vi "Control_giro_v2.vi"() -> ()   [LabVIEW 2025]
panel:
  in  "Boolean":bool
  out "Pulsos":dbl
  in  "B":bool
  in  "A":bool
  in  "stop":bool
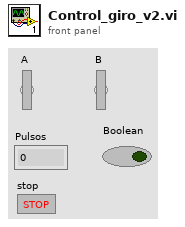
[diagram p1: front panel]
types:
  T1 = enum16{"Ini", "H1", "H2", "H3", "RES", "A1", "A2", "A3", "SUM"}
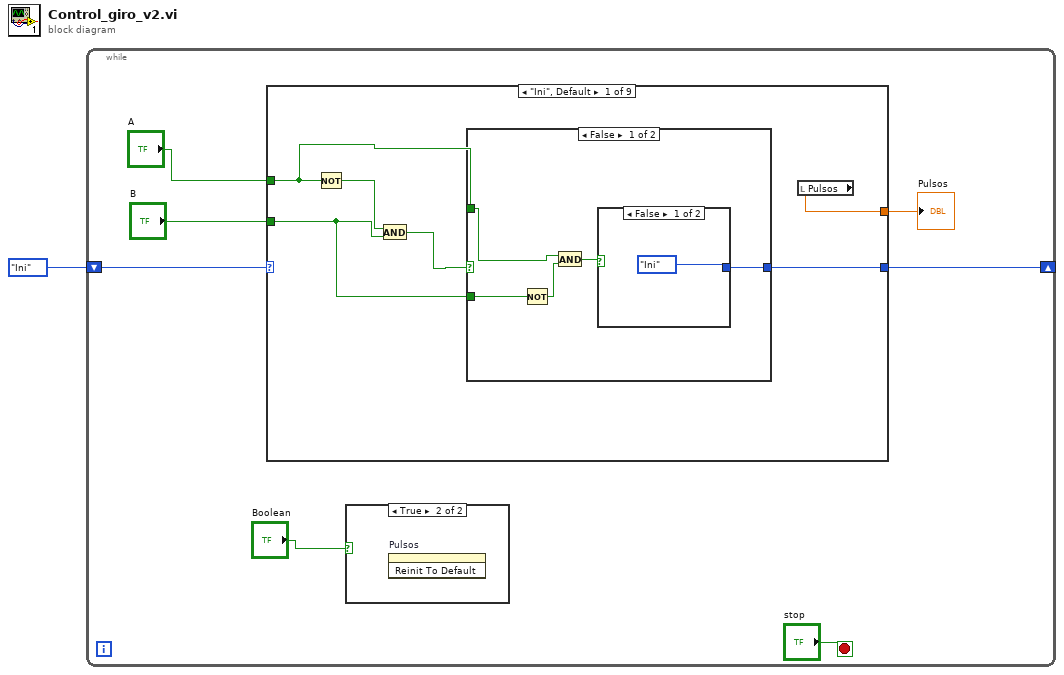
[diagram p0: block diagram]
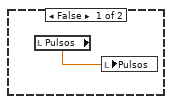
[diagram p2: hidden frame]
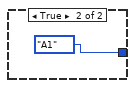
[diagram p3: hidden frame]
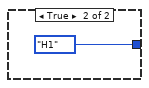
[diagram p4: hidden frame]
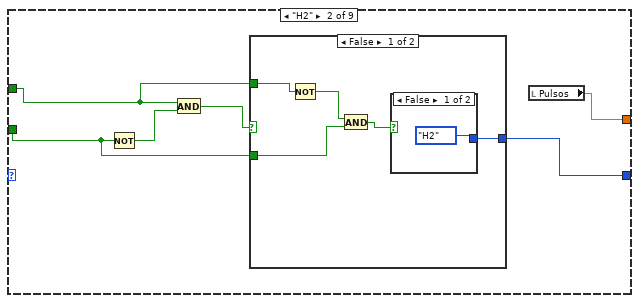
[diagram p5: hidden frame]
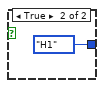
[diagram p6: hidden frame]
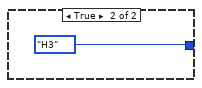
[diagram p7: hidden frame]
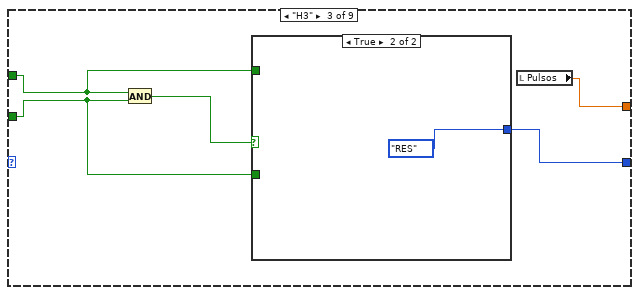
[diagram p8: hidden frame]
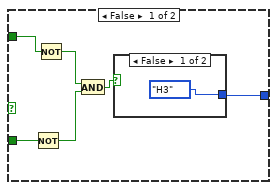
[diagram p9: hidden frame]
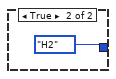
[diagram p10: hidden frame]
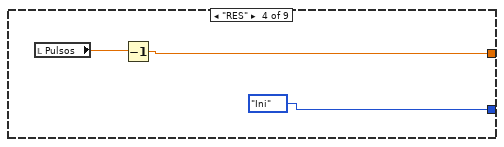
[diagram p11: hidden frame]
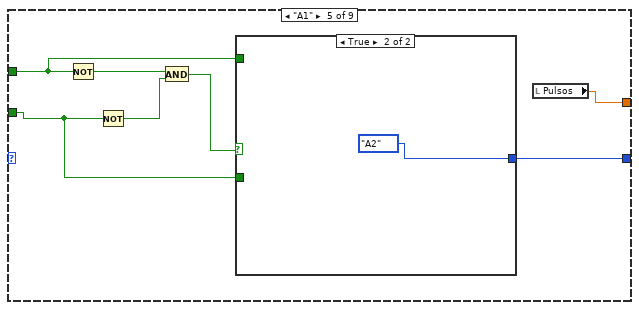
[diagram p12: hidden frame]
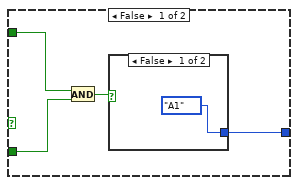
[diagram p13: hidden frame]
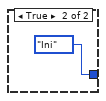
[diagram p14: hidden frame]
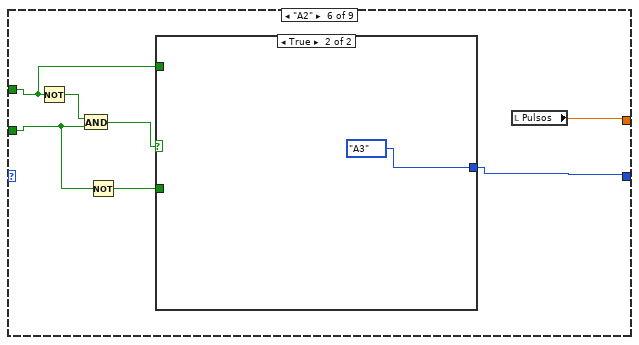
[diagram p15: hidden frame]
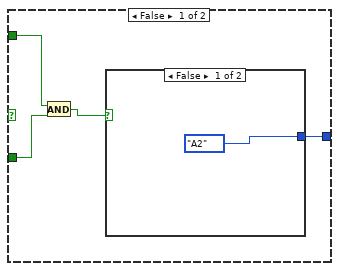
[diagram p16: hidden frame]
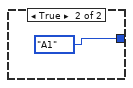
[diagram p17: hidden frame]
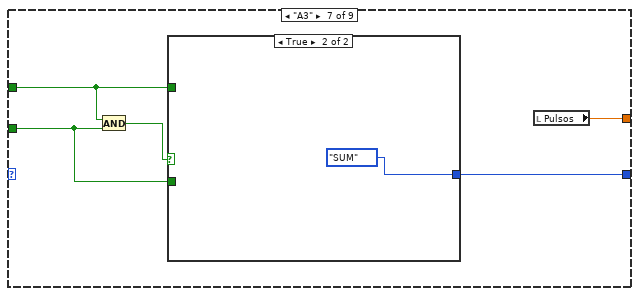
[diagram p18: hidden frame]
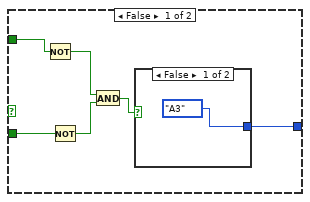
[diagram p19: hidden frame]
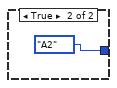
[diagram p20: hidden frame]
diagram:
  n1 = while {
    shift-right: [w4] -> _
    shift-left: T1."Ini" -> [w7]
    stop <- "stop" stop-if-true
    n2 = case shown="\"Ini\", Default" w7 {
      tunnel: "A" -> [w10 w27 w40 _ w57 w72 w84 _ w102]
      tunnel: "B" -> [w13 w26 w39 _ w56 w73 w85 _ w101]
      tunnel: [w14 w25 w41 T1."Ini" w58 w70 w86 T1."Ini" w103] -> w4
      tunnel: [w11 w24 w38 w53 w55 w69 w83 w98 w100] -> w3
      frame "Ini", Default {
        n3 = Not(x=w10) -> (.not. x?=w12:bool)
        n4 = And(x=w12, y=w13) -> (x .and. y?=w15:bool)
        n5 = case shown="False" w15 {
          tunnel: [w16 T1."H1"] -> w14
          tunnel: w13 -> [w20 _]
          tunnel: w10 -> [w19 _]
          frame False {
            n6 = Not(x=w20) -> (.not. x?=w18:bool)
            n7 = And(x=w19, y=w18) -> (x .and. y?=w17:bool)
            n8 = case shown="False" w17 {
              tunnel: [T1."Ini" T1."A1"] -> w16
              frame False {
              }
              frame True {
              }
            }
          }
          frame True {
          }
        }
        n9 = local read "Pulsos"() -> (w11:dbl)
      }
      frame "H2" {
        n10 = Not(x=w26) -> (.not. x?=w29:bool)
        n11 = And(x=w27, y=w29) -> (x .and. y?=w28:bool)
        n12 = case shown="False" w28 {
          tunnel: w27 -> [w34 _]
          tunnel: w26 -> [w33 _]
          tunnel: [w30 T1."H3"] -> w25
          frame False {
            n13 = Not(x=w34) -> (.not. x?=w32:bool)
            n14 = And(x=w32, y=w33) -> (x .and. y?=w31:bool)
            n15 = case shown="False" w31 {
              tunnel: [T1."H2" T1."H1"] -> w30
              frame False {
              }
              frame True {
              }
            }
          }
          frame True {
          }
        }
        n16 = local read "Pulsos"() -> (w24:dbl)
      }
      frame "H3" {
        n17 = And(x=w40, y=w39) -> (x .and. y?=w42:bool)
        n18 = case shown="True" w42 {
          tunnel: [w43 T1."RES"] -> w41
          tunnel: w40 -> [w48 _]
          tunnel: w39 -> [w47 _]
          frame False {
            n19 = Not(x=w47) -> (.not. x?=w44:bool)
            n20 = Not(x=w48) -> (.not. x?=w45:bool)
            n21 = And(x=w45, y=w44) -> (x .and. y?=w46:bool)
            n22 = case shown="False" w46 {
              tunnel: [T1."H3" T1."H2"] -> w43
              frame False {
              }
              frame True {
              }
            }
          }
          frame True {
          }
        }
        n23 = local read "Pulsos"() -> (w38:dbl)
      }
      frame "RES" {
        n24 = local read "Pulsos"() -> (w54:dbl)
        n25 = Decrement(x=w54) -> (x-1=w53:dbl)
      }
      frame "A1" {
        n26 = Not(x=w57) -> (.not. x?=w59:bool)
        n27 = Not(x=w56) -> (.not. x?=w61:bool)
        n28 = And(x=w59, y=w61) -> (x .and. y?=w60:bool)
        n29 = case shown="True" w60 {
          tunnel: [w63 T1."A2"] -> w58
          tunnel: w57 -> [w65 _]
          tunnel: w56 -> [w64 _]
          frame False {
            n30 = And(x=w65, y=w64) -> (x .and. y?=w62:bool)
            n31 = case shown="False" w62 {
              tunnel: [T1."A1" T1."Ini"] -> w63
              frame False {
              }
              frame True {
              }
            }
          }
          frame True {
          }
        }
        n32 = local read "Pulsos"() -> (w55:dbl)
      }
      frame "A2" {
        n33 = Not(x=w72) -> (.not. x?=w75:bool)
        n34 = And(x=w75, y=w73) -> (x .and. y?=w74:bool)
        n35 = Not(x=w73) -> (.not. x?=w71:bool)
        n36 = case shown="True" w74 {
          tunnel: w72 -> [w79 _]
          tunnel: w71 -> [w78 _]
          tunnel: [w76 T1."A3"] -> w70
          frame False {
            n37 = And(x=w79, y=w78) -> (x .and. y?=w77:bool)
            n38 = case shown="False" w77 {
              tunnel: [T1."A2" T1."A1"] -> w76
              frame False {
              }
              frame True {
              }
            }
          }
          frame True {
          }
        }
        n39 = local read "Pulsos"() -> (w69:dbl)
      }
      frame "A3" {
        n40 = And(x=w84, y=w85) -> (x .and. y?=w87:bool)
        n41 = case shown="True" w87 {
          tunnel: [w88 T1."SUM"] -> w86
          tunnel: w85 -> [w93 _]
          tunnel: w84 -> [w92 _]
          frame False {
            n42 = Not(x=w92) -> (.not. x?=w90:bool)
            n43 = Not(x=w93) -> (.not. x?=w89:bool)
            n44 = And(x=w90, y=w89) -> (x .and. y?=w91:bool)
            n45 = case shown="False" w91 {
              tunnel: [T1."A3" T1."A2"] -> w88
              frame False {
              }
              frame True {
              }
            }
          }
          frame True {
          }
        }
        n46 = local read "Pulsos"() -> (w83:dbl)
      }
      frame "SUM" {
        n47 = local read "Pulsos"() -> (w99:dbl)
        n48 = Increment(x=w99) -> (x+1=w98:dbl)
      }
      frame "H1" {
        n49 = Not(x=w101) -> (.not. x?=w105:bool)
        n50 = Not(x=w102) -> (.not. x?=w106:bool)
        n51 = And(x=w106, y=w105) -> (x .and. y?=w104:bool)
        n52 = case shown="True" w104 {
          tunnel: [w108 T1."H2"] -> w103
          tunnel: w102 -> [w110 _]
          tunnel: w101 -> [w109 _]
          frame False {
            n53 = And(x=w110, y=w109) -> (x .and. y?=w107:bool)
            n54 = case shown="False" w107 {
              tunnel: [T1."H1" T1."Ini"] -> w108
              frame False {
              }
              frame True {
              }
            }
          }
          frame True {
          }
        }
        n55 = local read "Pulsos"() -> (w100:dbl)
      }
    }
    "Pulsos" <- w3
    n56 = case shown="True" "Boolean" {
      frame False {
        n57 = local read "Pulsos"() -> (w9:dbl)
        n58 = local write "Pulsos"(w9) -> ()
      }
      frame True {
        n59 = invoke on="Pulsos" class="DigNum (strict)" method="Reinit To Default"() -> ()  [unwired: 3 in, 3 out]
      }
    }
  }
